vi "FollowBeeCircle.vi"(0 "Way Point X":dbl, 1 "Way Point Y":dbl, 2 "X Pos":dbl, 3 "Y Pos":dbl, 4 "Heading":dbl) -> (5 "Rudder Angle":dbl)   [LabVIEW 2014]
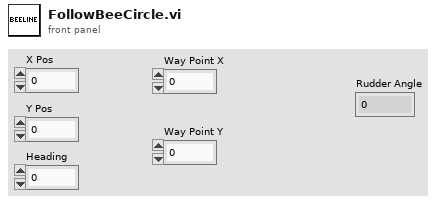
[diagram p1: front panel]
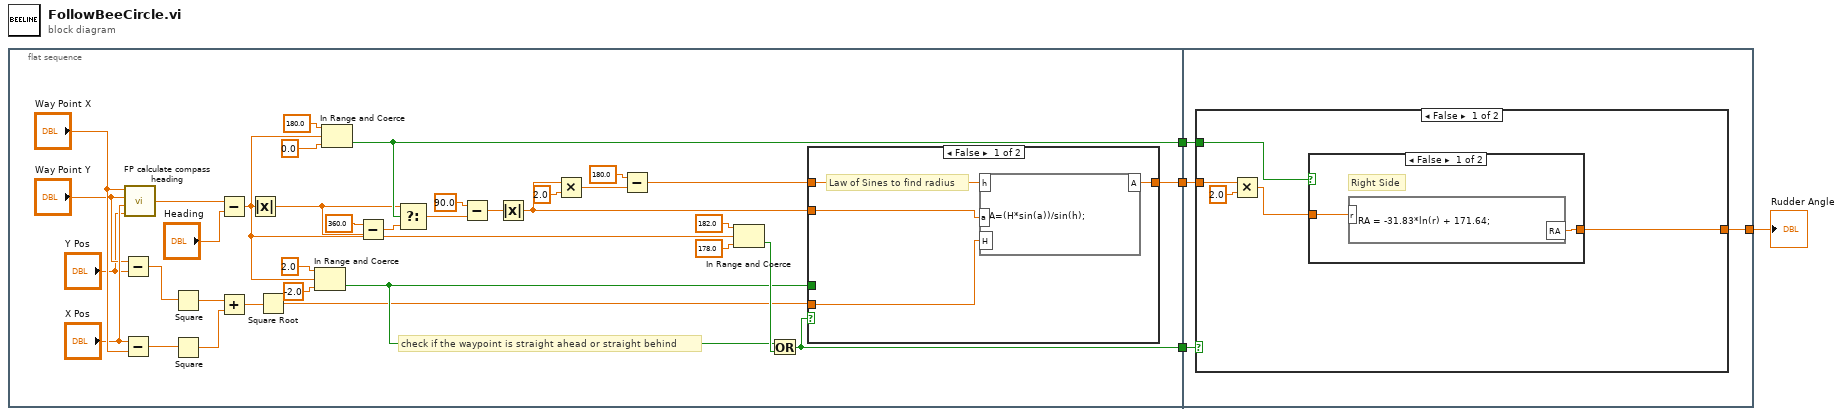
[diagram p0: block diagram]
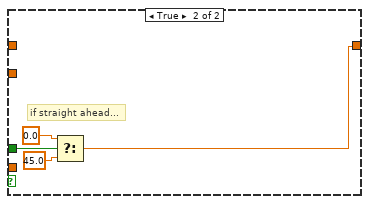
[diagram p2: hidden frame]
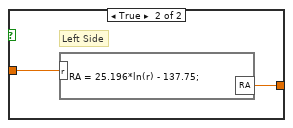
[diagram p3: hidden frame]
diagram:
  n1 = flat-sequence {
    tunnel: [w27] -> w4
    tunnel: [w17] -> w2
    tunnel: [w10] -> w1
    tunnel: w4 -> [w51]
    tunnel: [w49] -> w3
    tunnel: w2 -> [w50]
    tunnel: w1 -> [w48]
    frame #0 {
      # "check if the waypoint is straight ahead or straight behind"
      n2 = Subtract(x="Way Point Y", y="Y Pos") -> (x-y=w31:dbl)
      n3 = Subtract(x="X Pos", y="Way Point X") -> (x-y=w30:dbl)
      n4 = call "FP calculate compass heading.vi"("Y Location"="Y Pos", "X Location"="X Pos", "Waypoint Y"="Way Point Y", "Waypoint X"="Way Point X") -> ("Heading"=w39:dbl)
      n5 = Square(x=w31) -> (x^2=w28:dbl)
      n6 = Square(x=w30) -> (x^2=w29:dbl)
      n7 = Subtract(x=w39, y="Heading") -> (x-y=w5:dbl)
      n8 = Add(x=w28, y=w29) -> (x+y=w7:dbl)
      n9 = Absolute Value(x=w5) -> (abs(x)=w8:dbl)
      n10 = Square Root(x=w7) -> (sqrt(x)=w6:dbl)
      n11 = In Range and Coerce(upper limit=2.0 ("y"), x=w5, lower limit=-2.0 ("y")) -> (In Range?=w9:bool)  [unwired: 1 out]
      n12 = In Range and Coerce(upper limit=180.0, x=w5, lower limit=0.0) -> (In Range?=w27:bool)  [unwired: 1 out]
      n13 = Subtract(x=360.0 ("upper limit"), y=w8) -> (x-y=w16:dbl)
      n14 = Select(t=w8, s=w27, f=w16) -> (s? t:f=w24:dbl)
      n15 = Subtract(x=90.0 ("upper limit"), y=w24) -> (x-y=w23:dbl)
      n16 = Absolute Value(x=w23) -> (abs(x)=w19:dbl)
      n17 = Multiply(x=w19, y=2.0) -> (x*y=w20:dbl)
      n18 = Subtract(x=180.0 ("upper limit"), y=w20) -> (x-y=w18:dbl)
      n19 = In Range and Coerce(upper limit=182.0 ("y"), x=w5, lower limit=178.0 ("y")) -> (In Range?=w11:bool)  [unwired: 1 out]
      n20 = Or(x=w9, y=w11) -> (x .or. y?=w10:bool)
      n21 = case shown="False" w10 {
        tunnel: w6 -> [w40 _]
        tunnel: w19 -> [w43 _]
        tunnel: w18 -> [w42 _]
        tunnel: [w41 w46] -> w17
        tunnel: w9 -> [_ w44]
        frame False {
          # "Law of Sines to find radius"
          n22 = formula code="A=(H*sin(a))/sin(h);"("a"=w43, "H"=w40, "h"=w42) -> ("A"=w41:dbl)
        }
        frame True {
          # "if straight ahead..."
          n23 = Select(t=0.0, s=w44, f=45.0) -> (s? t:f=w46:dbl)
        }
      }
    }
    frame #1 {
      n24 = case shown="False" w48 {
        tunnel: w51 -> [w56 _]
        tunnel: w50 -> [w55 w61]
        tunnel: [w53 w61] -> w49
        frame False {
          n25 = Multiply(x=w55, y=2.0) -> (x*y=w52:dbl)
          n26 = case shown="False" w56 {
            tunnel: w52 -> [w58 w60]
            tunnel: [w57 w59] -> w53
            frame False {
              # "Right Side"
              n27 = formula code="RA = -31.83*ln(r) + 171.64;"("r"=w58) -> ("RA"=w57:dbl)
            }
            frame True {
              # "Left Side"
              n28 = formula code="RA = 25.196*ln(r) - 137.75;"("r"=w60) -> ("RA"=w59:dbl)
            }
          }
        }
        frame True {
          # "In this case, the waypoint is right ahead or right behind"
        }
      }
    }
  }
  "Rudder Angle" <- w3
